vi "GET.vi"(6 "timeout":i32=10000, 7 "output file":path, 8 "error in":errorcluster, 10 "url":string, 11 "Session In":refnum<class "Session.lvclass">) -> (0 "error out":errorcluster, 1 "body":string, 2 "headers":string, 3 "Session Out":refnum<class "Session.lvclass">, 4 "status code":u32)   [LabVIEW 2020, in "Library Commun.lvlib" / "Library Http.lvlib" / "Session.lvclass"]
doc: "Sends a web request that returns header and body data from a server, web page, or web service. This VI uses the GET HTTP method and does not submit any data to the server."
uses:
  Session.lvclass
  Session.lvclass/Session.ctl
  lvwebclient_32.dll
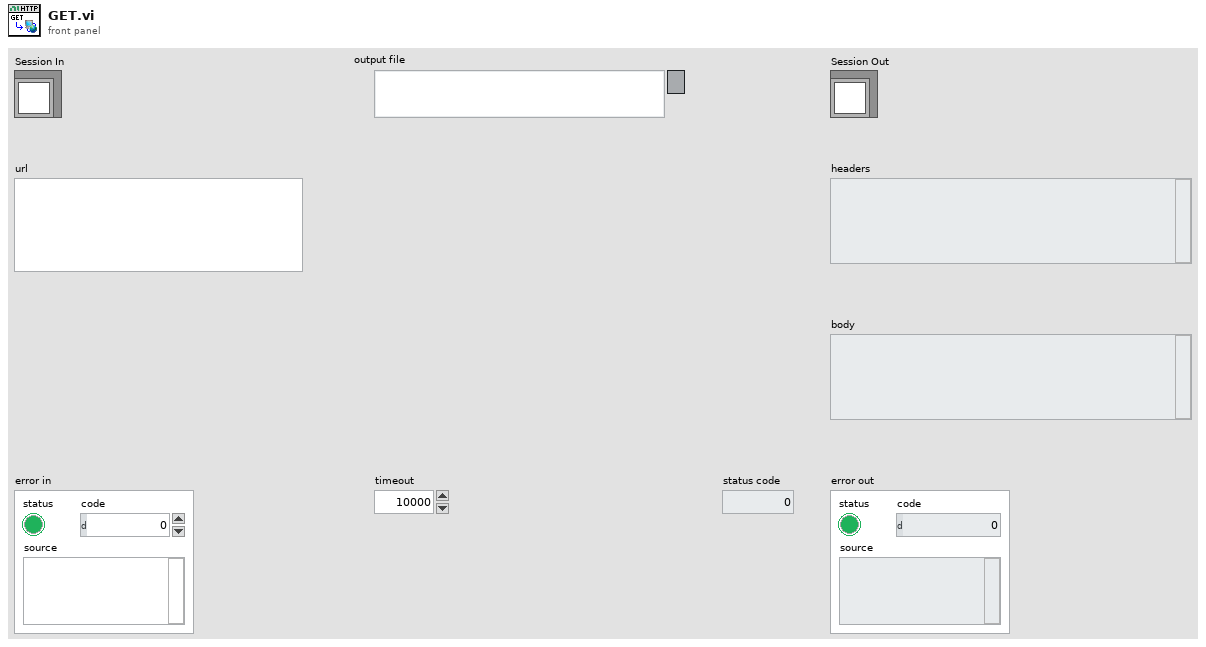
[diagram p1: front panel]
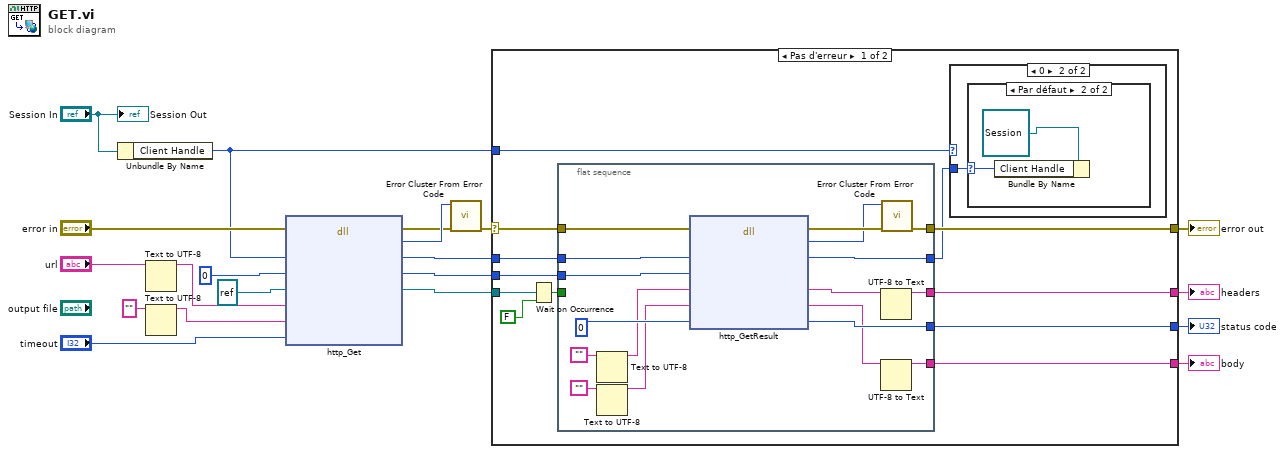
[diagram p0: block diagram]
diagram:
  n1 = Unbundle By Name("Session In") -> ("Client Handle"=w2:u32)
  n2 = Text to UTF-8(11:"url") -> (3:w14:string)  [unwired: 2 in, 1 out]
  n3 = Text to UTF-8(11:"" ("texte")) -> (3:w11:string)  [unwired: 2 in, 1 out]
  n4 = dll-call lib="C:/Users/ngarcin/OneDrive - Altyor/Standard TB/Class/Http Altyor/lvwebclient_*.*" fn="http_Get"(error in="error in", "handle"=w2, "request"=u32 0, "completeOccurrence"=refnum<k4> refnum ("occurrence"), "url"=w14, "outPath"=w11, "timeout"="timeout") -> (error out=w10:errorcluster, "return"=w18:i32, "handle"=w8:u32, "request"=w7:u32, "completeOccurrence"=w12:refnum<k4>)  [unwired: 5 in, 1 out]
  n5 = call <vilib>:"Error Cluster From Error Code.vi"("error in (no error)"=w10, "error code (0)"=w18) -> ("error out"=w20:errorcluster)  [unwired: 7 in]
  n6 = case shown="Pas d'erreur" w20 {
    selector: w20 -> [w30 w53]
    tunnel: w12 -> [w32 _]
    tunnel: w8 -> [w29 _]
    tunnel: w7 -> [w28 _]
    tunnel: [w27 _] -> w6
    tunnel: [w26 _] -> w5
    tunnel: [w25 _] -> w4
    tunnel: [w24 w53] -> w3
    tunnel: w2 -> [w23 _]
    frame No Error {
      n7 = Wait on Occurrence(1:FALSE, 2:w32) -> (0:w31:bool)  [unwired: 1 in]
      n8 = flat-sequence {
        tunnel: w31 -> [_]
        tunnel: w30 -> [w52]
        tunnel: w29 -> [w51]
        tunnel: w28 -> [w50]
        tunnel: [w48] -> w27
        tunnel: [w43] -> w26
        tunnel: [w42] -> w25
        tunnel: [w41] -> w24
        tunnel: [w40] -> w22
        frame #0 {
          n9 = Text to UTF-8(11:"") -> (3:w37:string)  [unwired: 2 in, 1 out]
          n10 = Text to UTF-8(11:"") -> (3:w36:string)  [unwired: 2 in, 1 out]
          n11 = dll-call lib="C:/Users/ngarcin/OneDrive - Altyor/Standard TB/Class/Http Altyor/lvwebclient_*.*" fn="http_GetResult"(error in=w52, "handle"=w51, "request"=w50, "returnHeader"=w37, "returnBody"=w36, "httpStatus"=u32 0) -> (error out=w47:errorcluster, "return"=w46:i32, "handle"=w40:u32, "returnHeader"=w45:string, "returnBody"=w44:string, "httpStatus"=w48:u32)  [unwired: 3 in, 1 out]
          n12 = UTF-8 to Text(11:w45) -> (3:w43:string)  [unwired: 2 in, 1 out]
          n13 = UTF-8 to Text(11:w44) -> (3:w42:string)  [unwired: 2 in, 1 out]
          n14 = call <vilib>:"Error Cluster From Error Code.vi"("error in (no error)"=w47, "error code (0)"=w46) -> ("error out"=w41:errorcluster)  [unwired: 7 in]
        }
      }
      n15 = case shown="0" w23 {
        tunnel: w22 -> [_ w33]
        frame Default {
        }
        frame 0 {
          n16 = case shown="Par défaut" w33 {
            selector: w33 -> [_ w35]
            frame 0 {
            }
            frame Default {
              n17 = Bundle By Name(cluster=refnum<class "Session.lvclass"> refnum ("Session Out"), "Client Handle"=w35) -> ()  [unwired: 1 out]
            }
          }
        }
      }
    }
    frame Error {
    }
  }
  "error out" <- w3
  "headers" <- w5
  "body" <- w4
  "status code" <- w6
  "Session Out" <- "Session In"
